vi "Configure LAN Trigger Output Line.vi"(0 "VISA resource name":refnum<visa-resource-name>, 1 "Connect State":bool=TRUE, 2 "IP Address":string="\"1.1.1.1\"", 5 "LAN Event Number (1)":u32=1 min=1 max=8 step=1, 7 "Trigger Logic Type":u16(ring) items=["Positive", "Negative"], 9 "Protocol":u16(ring) items=["TCP", "UDP", "Multicast"], 11 "error in (no error)":errorcluster, 12 "Stimulus Event":u16(ring) items=["None", "Front Pannel Trigger Key", "Notify Trigger Block 1", "Notify Trigger Block 2", "Notify Trigger Block 3", "Notify Trigger Block 4", "Notify Trigger Block 5", "Notify Trigger Block 6", "Notify Trigger Block 7", "Notify Trigger Block 8", "Command", "Digi IO Line 1", "Digi IO Line 2", "Digi IO Line 3", "Digi IO Line 4", "Digi IO Line 5", "Digi IO Line 6", "TSP-Link 1", "TSP-Link 2", "TSP-Link 3", "LAN 1", "LAN 2", "LAN 3", "LAN 4", "LAN 5", "LAN 6", "LAN 7", "LAN 8", "Blender 1", "Blender 2", "Timer 1", "Timer 2", "Timer 3", "Timer 4", "Analog Trigger", "External Trigger"]) -> (4 "VISA resource name out":refnum<visa-resource-name>, 15 "error out":errorcluster)   [LabVIEW 2018, in "Keithley DMM7512.lvlib"]
doc: "This VI sets the logic on which the trigger event detector and the output trigger generator operate on the given trigger line. Also sets the IP address, protocol type ans stimulus event."
uses:
  <instrlib>/Keithley DMM7512/Keithley DMM7512.lvlib
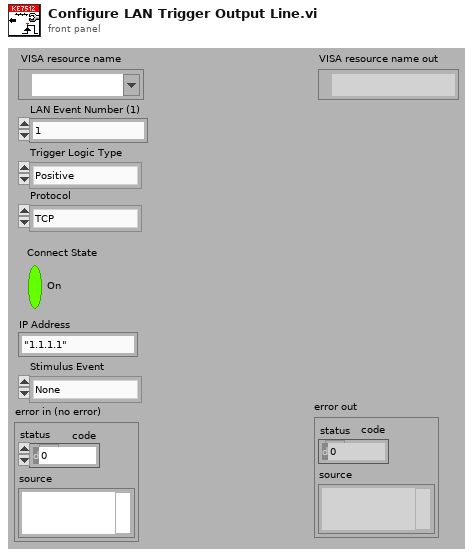
[diagram p1: front panel]
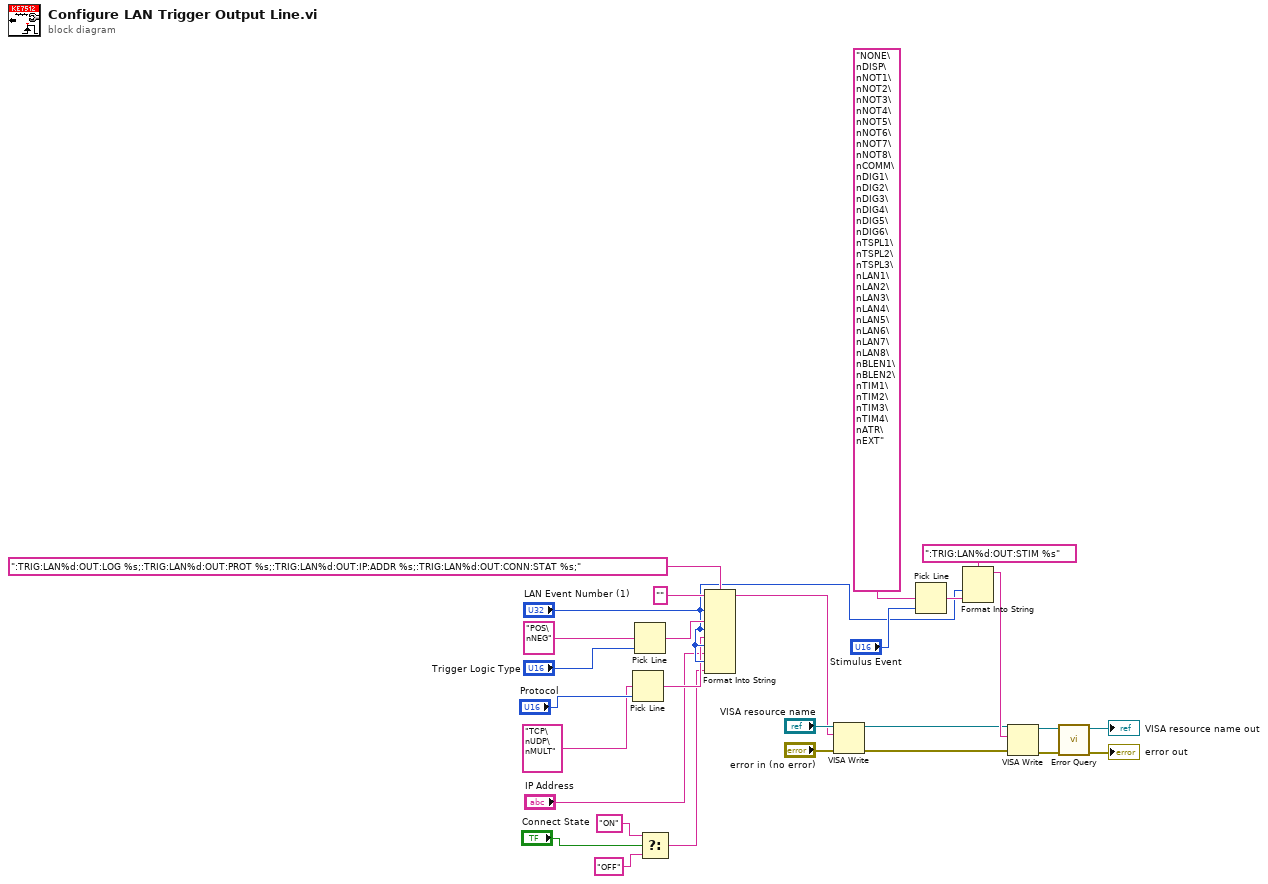
[diagram p0: block diagram]
diagram:
  n1 = Pick Line(multi-line string="TCP\nUDP\nMULT", line index="Protocol") -> (output string=w3:string)  [unwired: 1 in]
  n2 = Pick Line(multi-line string="POS\nNEG", line index="Trigger Logic Type") -> (output string=w19:string)  [unwired: 1 in]
  n3 = Select(t="ON" ("format string"), s="Connect State", f="OFF" ("format string")) -> (s? t:f=w1:string)
  n4 = Format Into String(format string=":TRIG:LAN%d:OUT:LOG %s;:TRIG:LAN%d:OUT:PROT %s;:TRIG:LAN%d:OUT:IP:ADDR %s;:TRIG:LAN%d:OUT:CONN:STAT %s;", initial string="", "LAN Event Number (1)", w19, "LAN Event Number (1)", w3, "LAN Event Number (1)", "IP Address", "LAN Event Number (1)", w1) -> (resulting string=w22:string)  [unwired: 1 in, 1 out]
  n5 = VISA Write(VISA resource name="VISA resource name", write buffer=w22, error in (no error)="error in (no error)") -> (VISA resource name out=w6:refnum<visa-resource-name>, error out=w5:errorcluster)  [unwired: 1 out]
  n6 = Pick Line(multi-line string="NONE\nDISP\nNOT1\nNOT2\nNOT3\nNOT4\nNOT5\nNOT6\nNOT7\nNOT8\nCOMM\nDIG1\nDIG2\nDIG3\nDIG4\nDIG5\nDIG6\nTSPL1\nTSPL2\nTSPL3\nLAN1\nLAN2\nLAN3\nLAN4\nLAN5\nLAN6\nLAN7\nLAN8\nBLEN1\nBLEN2\nTIM1\nTIM2\nTIM3\nTIM4\nATR\nEXT", line index="Stimulus Event") -> (output string=w16:string)  [unwired: 1 in]
  n7 = Format Into String(format string=":TRIG:LAN%d:OUT:STIM %s", "LAN Event Number (1)", w16) -> (resulting string=w12:string)  [unwired: 2 in, 1 out]
  n8 = VISA Write(VISA resource name=w6, write buffer=w12, error in (no error)=w5) -> (VISA resource name out=w13:refnum<visa-resource-name>, error out=w14:errorcluster)  [unwired: 1 out]
  n9 = call <instrlib>:"Error Query.vi"("error in (no error)"=w14, "VISA resource name"=w13) -> ("error out"=→"error out":errorcluster, "VISA resource name out"=→"VISA resource name out":refnum<visa-resource-name>)  [unwired: 8 out]
